vi "GetMatlabTempParamData.vi"(10 "index":dbl, 11 "ExpID":string) -> (3 "Matlab param data":T1[](array[typedef]))   [LabVIEW 2017]
uses:
  Types/MatlabDataBundle.ctl
  Types/MatlabDataType.ctl
  Types/MatlabDataContainerType.ctl
panel:
  out "Param Data before convert":T1[](array[typedef])
  in  "Clear Temp?":bool=TRUE
  out "error out":errorcluster
  in  "error in":errorcluster
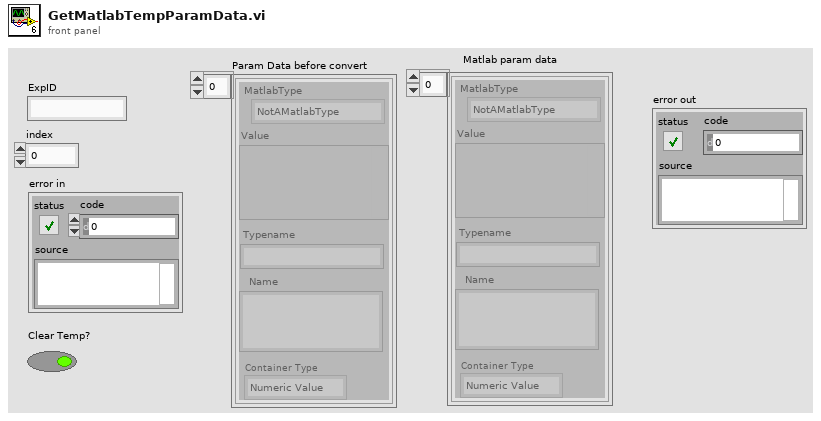
[diagram p1: front panel]
types:
  T1 = typedef "MatlabDataBundle.ctl" = cluster{"MatlabType":T2, "Value":variant, "Name":string, "Typename":string, "Container Type":T3}
  T2 = typedef "MatlabDataType.ctl" = enum16{"NotAMatlabType", "Real", "Complex", "String", "Boolean"}
  T3 = typedef "MatlabDataContainerType.ctl" = enum16{"Numeric Value", "Numeric Array", "Waveform"}
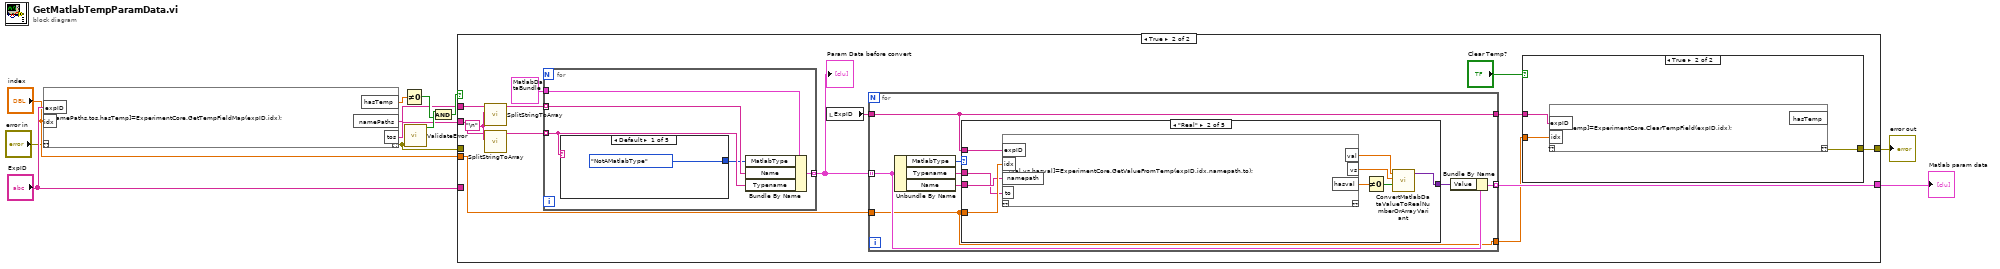
[diagram p0: block diagram]
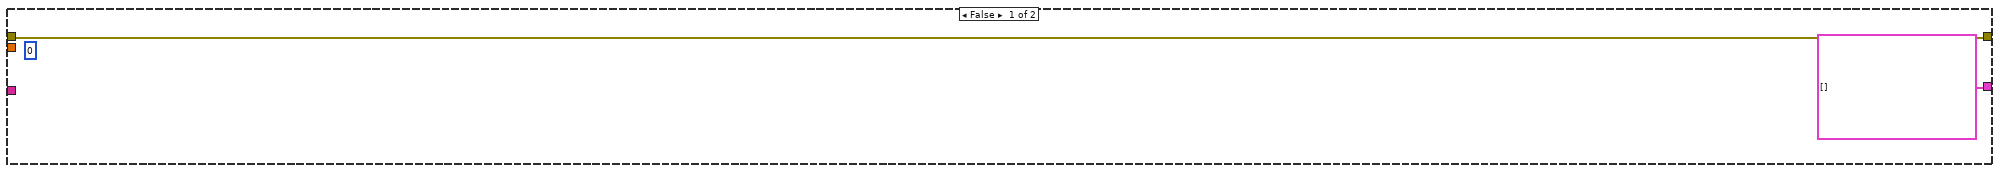
[diagram p2: hidden frame]
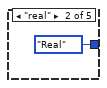
[diagram p3: hidden frame]
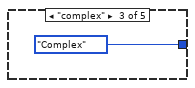
[diagram p4: hidden frame]
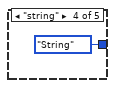
[diagram p5: hidden frame]
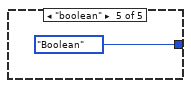
[diagram p6: hidden frame]
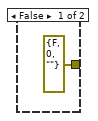
[diagram p7: hidden frame]
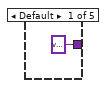
[diagram p8: hidden frame]
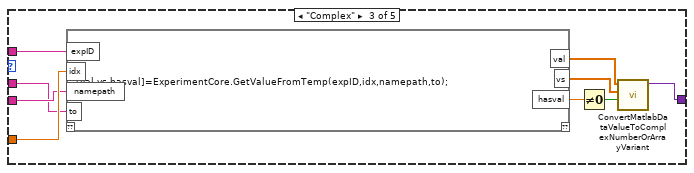
[diagram p9: hidden frame]
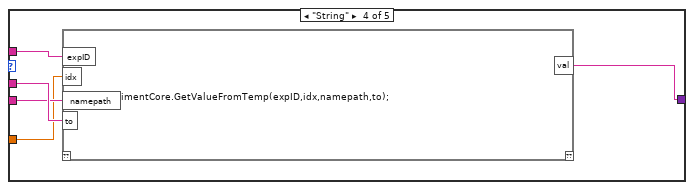
[diagram p10: hidden frame]
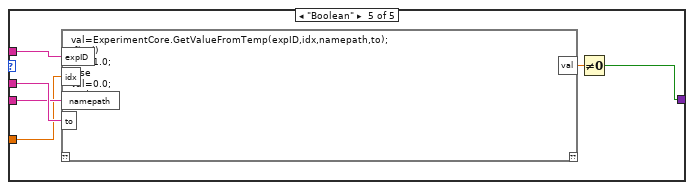
[diagram p11: hidden frame]
diagram:
  n1 = script code="[namePaths,tos,hasTemp]=ExperimentCore.GetTempFieldMap(expID,idx);"("??"="error in", "expID"="ExpID", "idx"="index") -> ("??"=w8:errorcluster, "hasTemp"=w11:dbl, "namePaths"=w1:string, "tos"=w2:string)
  n2 = Not Equal To 0?(x=w11) -> (x != 0?=w6:bool)
  n3 = call "ValidateError.vi"("error in (no error)"=w8) -> ("NoError?"=w7:bool)  [unwired: 9 in, 1 out]
  n4 = And(x=w7, y=w6) -> (x .and. y?=w5:bool)
  n5 = case shown="True" w5 {
    tunnel: [T1[] [] w28] -> w12
    tunnel: "ExpID" -> [_ _]
    tunnel: "index" -> [_ w27]
    tunnel: w8 -> [w13 _]
    tunnel: [w13 w16] -> w3
    tunnel: w2 -> [_ w21]
    tunnel: w1 -> [_ w20]
    frame False {
      (unwired) 0
    }
    frame True {
      w22 = "\n"
      n6 = call "SplitStringToArray.vi"("search string/char (-)"=w22, "String in"=w20) -> ("Split(s)"=w24:string[])  [unwired: 9 in]
      n7 = call "SplitStringToArray.vi"("search string/char (-)"=w22, "String in"=w21) -> ("Split(s)"=w25:string[])  [unwired: 9 in]
      n8 = for {
        tunnel: w24 -> [w32] mode=indexing
        tunnel: w25 -> [w30] mode=indexing
        tunnel: T1 {"MatlabType"=enum."NotAMatlabType", "Value"=variant, "Name"="", "Typename"="", "Container Type"=enum."Numeric Value"} ("MatlabDataBundle") -> [w33]
        tunnel: [w31] -> w19 mode=indexing
        n9 = case shown="Default" w30 {
          tunnel: [MatlabDataType."NotAMatlabType" ("MatlabType") MatlabDataType."Real" ("MatlabType") MatlabDataType."Complex" ("MatlabType") MatlabDataType."String" ("MatlabType") MatlabDataType."Boolean" ("MatlabType")] -> w29
          frame Default {
          }
          frame "real" {
          }
          frame "complex" {
          }
          frame "string" {
          }
          frame "boolean" {
          }
        }
        n10 = Bundle By Name(cluster=w33, "MatlabType"=w29, "Name"=w32, "Typename"=w30) -> (w31:T1)
      }
      "Param Data before convert" <- w19
      n11 = local read "ExpID"() -> (w18:string)
      n12 = for {
        tunnel: w19 -> [w47] mode=indexing
        tunnel: [w46] -> w28 mode=indexing
        tunnel: w27 -> [w43]
        tunnel: w18 -> [w44]
        tunnel: [w44] -> w17
        tunnel: [w43] -> w15
        n13 = Unbundle By Name(w47) -> ("MatlabType"=w45:T2, "Typename"=w50:string, "Name"=w49:string)
        n14 = case shown="\"Real\"" w45 {
          tunnel: [variant ("Reshaped VArray") w55 w61 w74 w79] -> w48
          tunnel: w44 -> [_ w60 w69 w73 w78]
          tunnel: w50 -> [_ w57 w66 w72 w77]
          tunnel: w49 -> [_ w58 w67 w71 w76]
          tunnel: w43 -> [_ w59 w68 w70 w75]
          frame Default {
          }
          frame "Real" {
            n15 = script code="[val,vs,hasval]=ExperimentCore.GetValueFromTemp(expID,idx,namepath,to);"("expID"=w60, "idx"=w59, "to"=w57, "namepath"=w58) -> ("val"=w56:dbl[], "vs"=w53:dbl[], "hasval"=w54:dbl)  [unwired: 1 in, 1 out]
            n16 = Not Equal To 0?(x=w54) -> (x != 0?=w52:bool)
            n17 = call "ConvertMatlabDataValueToRealNumberOrArrayVariant.vi"("Has Value"=w52, "Sizes"=w53, "Data"=w56) -> ("Reshaped VArray"=w55:variant)  [unwired: 8 in]
          }
          frame "Complex" {
            n18 = script code="[val,vs,hasval]=ExperimentCore.GetValueFromTemp(expID,idx,namepath,to);"("expID"=w69, "idx"=w68, "to"=w66, "namepath"=w67) -> ("val"=w65:cdb[], "vs"=w64:dbl[], "hasval"=w63:dbl)  [unwired: 1 in, 1 out]
            n19 = Not Equal To 0?(x=w63) -> (x != 0?=w62:bool)
            n20 = call "ConvertMatlabDataValueToComplexNumberOrArrayVariant.vi"("Has Value"=w62, "Sizes"=w64, "Data"=w65) -> ("Reshaped VArray"=w61:variant)  [unwired: 8 in]
          }
          frame "String" {
            n21 = script code="val=ExperimentCore.GetValueFromTemp(expID,idx,namepath,to);"("expID"=w73, "idx"=w70, "namepath"=w71, "to"=w72) -> ("val"=w74:string)  [unwired: 1 in, 1 out]
          }
          frame "Boolean" {
            n22 = script code="val=ExperimentCore.GetValueFromTemp(expID,idx,namepath,to);\nif(val)\nval=1.0;\nelse\nval=0.0;\nend"("expID"=w78, "idx"=w75, "namepath"=w76, "to"=w77) -> ("val"=w80:dbl)  [unwired: 1 in, 1 out]
            n23 = Not Equal To 0?(x=w80) -> (x != 0?=w79:bool)
          }
        }
        n24 = Bundle By Name(cluster=w47, "Value"=w48) -> (w46:T1)
      }
      n25 = case shown="True" "Clear Temp?" {
        tunnel: w17 -> [_ w42]
        tunnel: w15 -> [_ w41]
        tunnel: [errorcluster {"status"=FALSE, "code"=0, "source"=""} ("error IO") w40] -> w16
        frame False {
        }
        frame True {
          n26 = script code="[hasTemp]=ExperimentCore.ClearTempField(expID,idx);"("expID"=w42, "idx"=w41) -> ("??"=w40:errorcluster)  [unwired: 1 in, 1 out]
        }
      }
    }
  }
  "Matlab param data" <- w12
  "error out" <- w3
